vi "实时小时数据单参数上传.vi"(11 "错误输入（无错误）":errorcluster) -> (4 "数据发送起始时间":timestamp format="%<%.3X\n%Y/%m/%d>T", 15 "error out":errorcluster)   [LabVIEW 2016, in "数据传输系统.lvlib"]
uses:
  <vilib>/Utility/config.llb/Read Key (String).vi
  <vilib>/Utility/config.llb/Write Key (String).vi
  <vilib>/Utility/config.llb/NI_LVConfig.lvlib
panel:
  out "数据拆分":bool
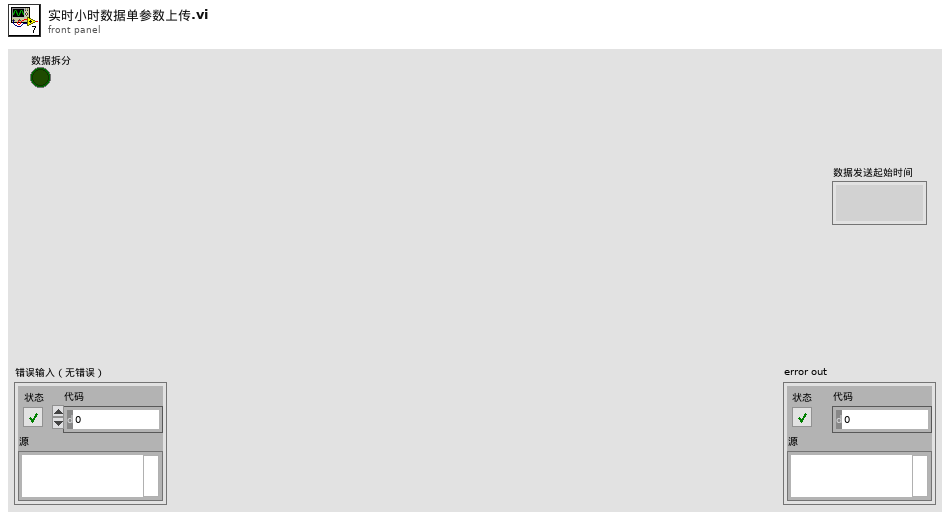
[diagram p1: front panel]
types:
  T1 = cluster{"CODMn":string, "CODCr":string, "DO":string, "铜":string, "PH":string, "氨氮":string, "比电导率":string, "水温":string, "COD":string, "浊度":string, "总氮":string, "总磷":string, "叶绿素a":string, "藻密度":string, "水位":string, "流速":string, "瞬时流量":string, "累积流量":string, "亚硝酸盐":string, "硫化物":string, "ORP":string, "铅":string, "镉":string, "锌":string, "镍":string, "锰":string, "汞":string, "气温":string, "气压":string, "风速":string, "风向":string, "盐度":string, "磷酸盐":string, "硝氮":string, "氟化物":string, "挥发酚":string, "氯化物":string, "蓝绿藻":string}
  T2 = cluster{"setini":string, "sysini":string, "hechaini":string, "actualwrite":string, "actualread":string, "datasent":string, "反控命令信息队列":string, "反控与仪器交互":string}
  T3 = typedef "NI_LVConfig.lvlib/Config Data RefNum.ctl" = refnum<k1>
  T4 = cluster{"time1":string, "time2":string, "time3":string, "time4":string, "time5":string, "time6":string, "time7":string, "time8":string, "time9":string, "time10":string, "time11":string, "time12":string, "time13":string, "time14":string, "time15":string, "time16":string, "time17":string, "time18":string, "time19":string, "time20":string, "time21":string, "time22":string, "time23":string, "time24":string, "time25":string, "time26":string, "time27":string, "time28":string, "time29":string, "time30":string, "time31":string, "time32":string, "time33":string, "time34":string, "time35":string, "time36":string, "time37":string, "time38":string}
  T5 = cluster{"水样数据索引[0]":string, "水样数据索引[1]":string, "水样数据索引[2]":string, "水样数据索引[3]":string, "水样数据索引[4]":string, "水样数据索引[5]":string, "水样数据索引[6]":string, "水样数据索引[7]":string, "水样数据索引[8]":string, "水样数据索引[9]":string, "水样数据索引[10]":string, "水样数据索引[11]":string, "水样数据索引[12]":string, "水样数据索引[13]":string, "水样数据索引[14]":string, "水样数据索引[15]":string, "水样数据索引[16]":string, "水样数据索引[17]":string, "水样数据索引[18]":string, "水样数据索引[19]":string, "水样数据索引[20]":string, "水样数据索引[21]":string, "水样数据索引[22]":string, "水样数据索引[23]":string, "水样数据索引[24]":string, "水样数据索引[25]":string, "水样数据索引[26]":string, "水样数据索引[27]":string, "水样数据索引[28]":string, "水样数据索引[29]":string, "水样数据索引[30]":string, "水样数据索引[31]":string, "水样数据索引[32]":string, "水样数据索引[33]":string, "水样数据索引[34]":string, "水样数据索引[35]":string, "水样数据索引[36]":string, "水样数据索引[37]":string}
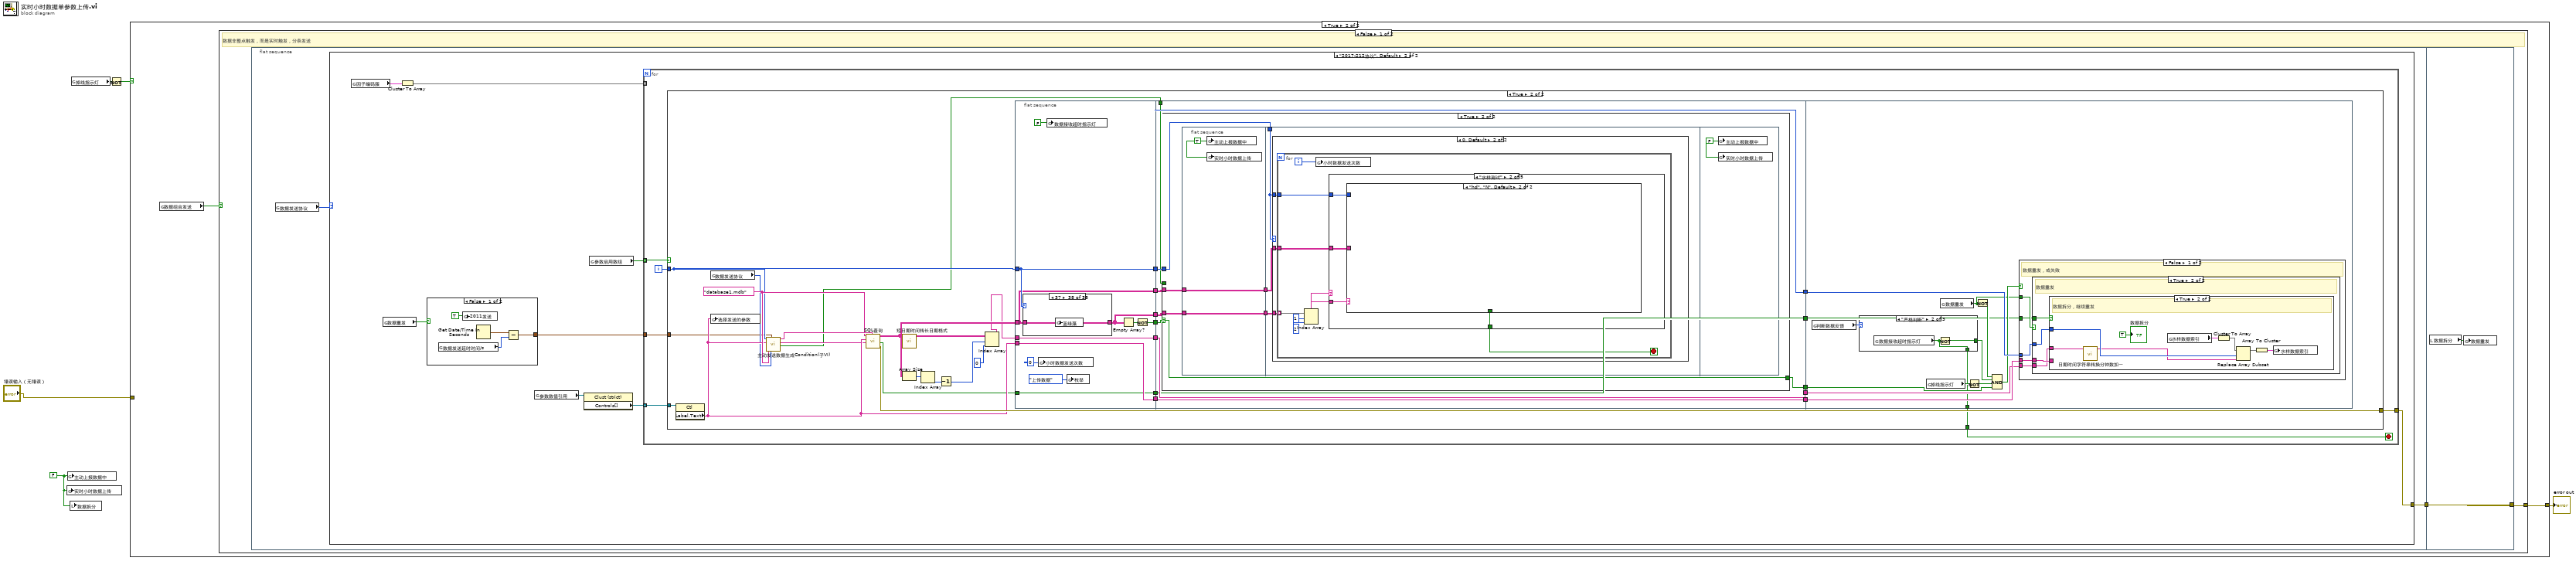
[diagram p0: block diagram]
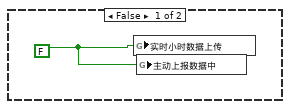
[diagram p2: hidden frame]
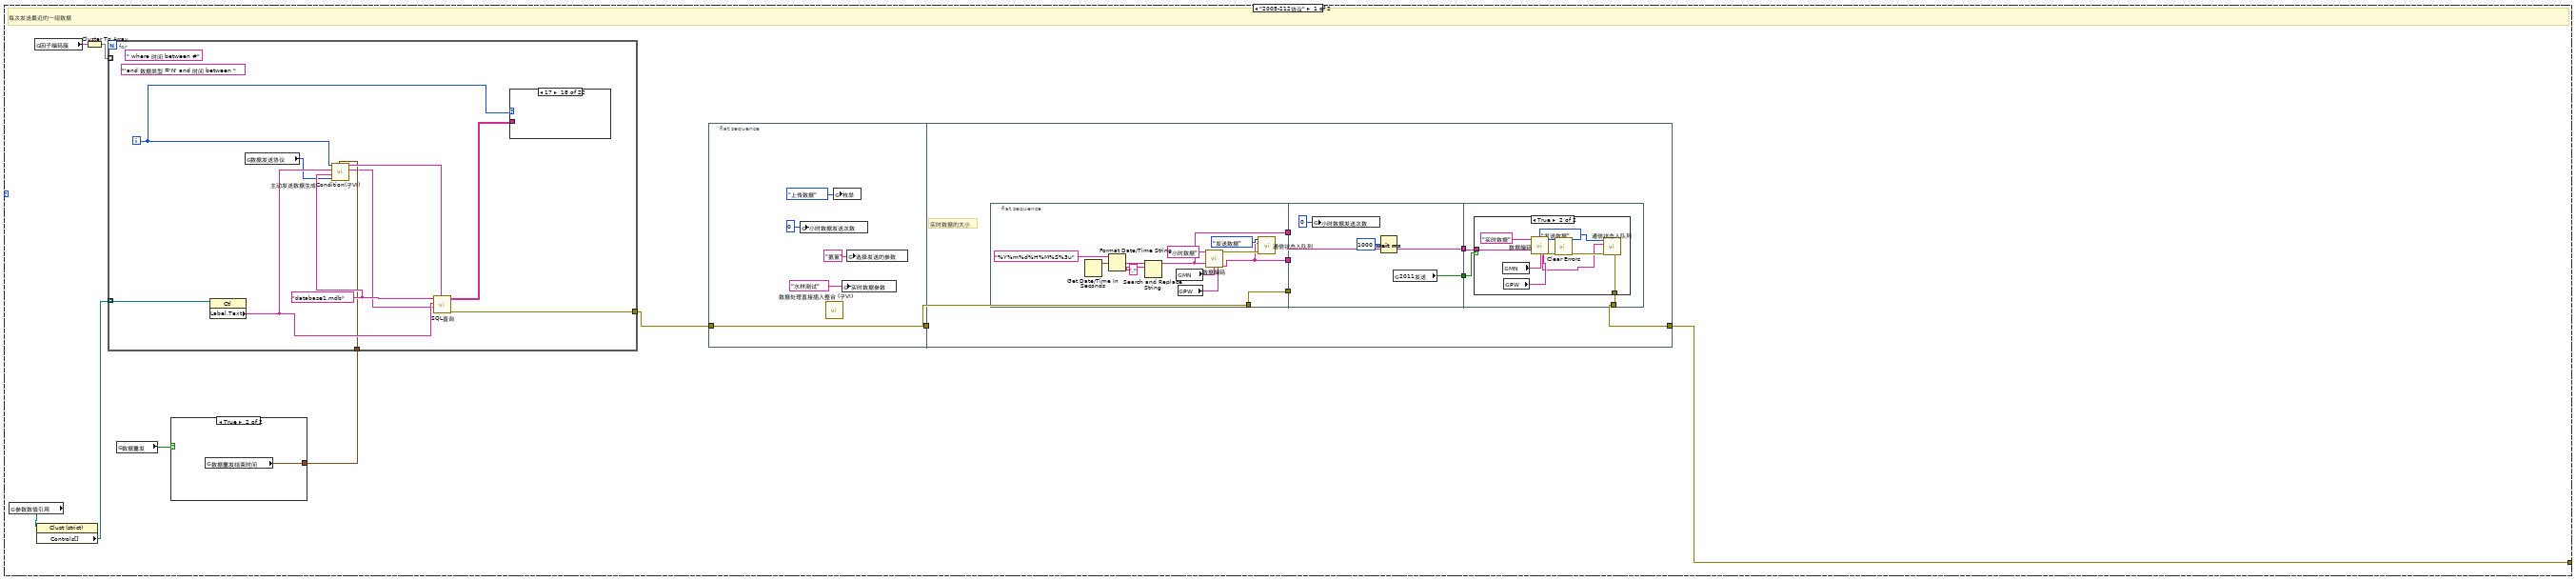
[diagram p3: hidden frame]
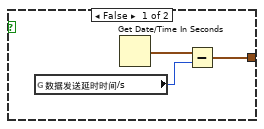
[diagram p4: hidden frame]
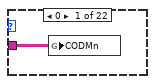
[diagram p6: hidden frame]
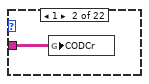
[diagram p7: hidden frame]
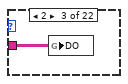
[diagram p8: hidden frame]
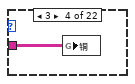
[diagram p9: hidden frame]
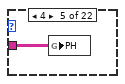
[diagram p10: hidden frame]
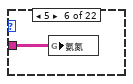
[diagram p11: hidden frame]
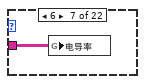
[diagram p12: hidden frame]
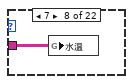
[diagram p13: hidden frame]
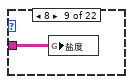
[diagram p14: hidden frame]
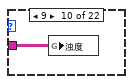
[diagram p15: hidden frame]
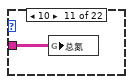
[diagram p16: hidden frame]
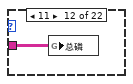
[diagram p17: hidden frame]
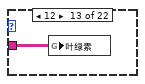
[diagram p18: hidden frame]
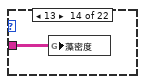
[diagram p19: hidden frame]
diagram:
  w1 = FALSE ("小时数据上传")
  n1 = global write "全局1.vi" "实时小时数据上传"(w1) -> ()
  n2 = global write "全局 数据发送重叠.vi" "主动上报数据中"(w1) -> ()
  n3 = local write "数据拆分"(w1) -> ()
  n4 = global read "全局 数据发送重叠.vi" "掉线指示灯"() -> (w5:bool)
  n5 = Not(x=w5) -> (.not. x?=w4:bool)
  n6 = case shown="True" w4 {
    tunnel: [_ w8] -> w3
    tunnel: "错误输入（无错误）" -> [_ _]
    frame False {
      w6 = FALSE ("小时数据上传")
      n7 = global write "全局1.vi" "实时小时数据上传"(w6) -> ()
      n8 = global write "全局 数据发送重叠.vi" "主动上报数据中"(w6) -> ()
    }
    frame True {
      n9 = global read "断电保存全局.vi" "数据组合发送"() -> (w7:bool)
      n10 = case shown="False" w7 {
        tunnel: [w9 _] -> w8
        frame False {
          # "数据非整点触发，而是实时触发，分条发送"
          n11 = flat-sequence {
            tunnel: [w12] -> w10
            tunnel: [w371] -> w9
            tunnel: w10 -> [w371]
            frame #0 {
              n12 = global read "断电保存全局.vi" "数据发送协议"() -> (w11:enum16{"2005-212协议", "2017-212协议"})
              n13 = case shown="\"2017-212协议\", Default" w11 {
                tunnel: [w17 w99] -> w12
                frame "2005-212协议" {
                  # "每次发送最近的一组数据"
                  n14 = global read "断电保存全局.vi" "参数数值引用"() -> (w15:refnum<vi>)
                  n15 = global read "断电保存全局.vi" "因子编码簇"() -> (w16:T1)
                  n16 = property class="Clust (strict)"(reference=w15) -> ("Controls[]"=w18:refnum<vi>[])  [unwired: 1 in, 2 out]
                  n17 = Cluster To Array(cluster=w16) -> (array=w21:string[])
                  n18 = global read "断电保存全局.vi" "数据重发"() -> (w14:bool)
                  n19 = case shown="True" w14 {
                    tunnel: [w22 w25] -> w13
                    frame False {
                      n20 = global read "断电保存全局.vi" "数据发送延时时间/s"() -> (w23:i32)
                      n21 = Get Date/Time In Seconds() -> (seconds since 1Jan1904=w24:timestamp)
                      n22 = Subtract(x=w24, y=w23) -> (x-y=w22:timestamp)
                    }
                    frame True {
                      n23 = global read "断电保存全局.vi" "数据重发结束时间"() -> (w25:timestamp)
                    }
                  }
                  n24 = for {
                    tunnel: w21 -> [_] mode=indexing
                    tunnel: [w75] -> w20
                    tunnel: w18 -> [w70] mode=indexing
                    tunnel: w13 -> [w67]
                    i -> [w68]
                    (unwired) " where 时间 between #"
                    w73 = "database1.mdb" ("database")
                    (unwired) "'and 数据类型 ='N' and 时间 between "
                    n25 = property class="Ctl"(reference=w70) -> ("Label.Text"=w74:string)  [unwired: 1 in, 2 out]
                    n26 = global read "断电保存全局.vi" "数据发送协议"() -> (w71:enum16{"2005-212协议", "2017-212协议"})
                    n27 = call "主动发送数据生成Condition(子VI).vi"("结束时间"=w67, "数据发送协议"=w71, "database"=w73, "Label.Text"=w74, "数值"=w68) -> ("columns"=w66:string[], "CONDITION"=w72:string)  [unwired: 3 in, 2 out]
                    n28 = call "SQL查询.vi"("condition"=w72, "columns"=w66, "table输入"=w74, "database"=w73) -> ("error out"=w75:errorcluster, "data"=w69:string[][])  [unwired: 4 in, 2 out]
                    n29 = case shown="17" w68 {
                      tunnel: w69 -> [w76 w77 w78 w79 w80 w81 w82 w83 w84 w85 w86 w87 w88 w89 _ _ _ _ w90 w91 w92 _]
                      frame 0 {
                        n30 = global write "全局 所有参数.vi" "CODMn"(w76) -> ()
                      }
                      frame 1 {
                        n31 = global write "全局 所有参数.vi" "CODCr"(w77) -> ()
                      }
                      frame 2 {
                        n32 = global write "全局 所有参数.vi" "DO"(w78) -> ()
                      }
                      frame 3 {
                        n33 = global write "全局 所有参数.vi" "铜"(w79) -> ()
                      }
                      frame 4 {
                        n34 = global write "全局 所有参数.vi" "PH"(w80) -> ()
                      }
                      frame 5 {
                        n35 = global write "全局 所有参数.vi" "氨氮"(w81) -> ()
                      }
                      frame 6 {
                        n36 = global write "全局 所有参数.vi" "电导率"(w82) -> ()
                      }
                      frame 7 {
                        n37 = global write "全局 所有参数.vi" "水温"(w83) -> ()
                      }
                      frame 8 {
                        n38 = global write "全局 所有参数.vi" "盐度"(w84) -> ()
                      }
                      frame 9 {
                        n39 = global write "全局 所有参数.vi" "浊度"(w85) -> ()
                      }
                      frame 10 {
                        n40 = global write "全局 所有参数.vi" "总氮"(w86) -> ()
                      }
                      frame 11 {
                        n41 = global write "全局 所有参数.vi" "总磷"(w87) -> ()
                      }
                      frame 12 {
                        n42 = global write "全局 所有参数.vi" "叶绿素"(w88) -> ()
                      }
                      frame 13 {
                        n43 = global write "全局 所有参数.vi" "藻密度"(w89) -> ()
                      }
                      frame 14 {
                      }
                      frame 15 {
                      }
                      frame 16 {
                      }
                      frame 17 {
                      }
                      frame 18 {
                        n44 = global write "全局 所有参数.vi" "亚硝酸盐"(w90) -> ()
                      }
                      frame 19 {
                        n45 = global write "全局 所有参数.vi" "硫化物"(w91) -> ()
                      }
                      frame 20 {
                        n46 = global write "全局 所有参数.vi" "ORP"(w92) -> ()
                      }
                      frame 21, Default {
                      }
                    }
                  }
                  n47 = flat-sequence {
                    tunnel: w20 -> [w26]
                    tunnel: [w26] -> w19
                    tunnel: w19 -> [w35]
                    tunnel: [w34] -> w17
                    frame #0 {
                      n48 = global write "全局 小时数据发送次数.vi" "小时数据发送次数"(0 ("小时数据发送次数")) -> ()
                      n49 = call "数据处理直接插入整合 (子VI).vi"() -> ()  [unwired: 12 in]
                      n50 = global write "全局1.vi" "枚举"(enum16{"返回请求应答", "上传数据", "返回执行结果"}."上传数据" ("枚举")) -> ()
                      n51 = global write "全局 实时数据参数.vi" "实时数据参数"("水样测试" ("实时数据参数")) -> ()
                      n52 = global write "全局 水样时间.vi" "选择发送的参数"("氨氮" ("选择发送的参数")) -> ()
                    }
                    frame #1 {
                      # "实时数据的大小"
                      n53 = flat-sequence {
                        tunnel: [w38] -> w37
                        tunnel: [w41] -> w36
                        tunnel: w35 -> [w41]
                        tunnel: [w40] -> w33
                        tunnel: w37 -> [_]
                        tunnel: w36 -> [_]
                        tunnel: w33 -> [w51]
                        tunnel: [w51] -> w32
                        tunnel: [w50] -> w31
                        tunnel: [w56] -> w34
                        tunnel: w32 -> [w55]
                        tunnel: w31 -> [w54]
                        frame #0 {
                          n54 = Get Date/Time In Seconds() -> (seconds since 1Jan1904=w47:timestamp)
                          n55 = Format Date/Time String(time format string (%c)="%Y%m%d%H%M%S%3u" ("时间格式字符串(%c)"), seconds (now)=w47) -> (date/time string=w48:string)  [unwired: 1 in]
                          n56 = Search and Replace String(input string=w48, search string="." ("搜索字符串")) -> (result string=w40:string)  [unwired: 6 in, 3 out]
                          n57 = global read "断电保存全局.vi" "MN"() -> (w44:string)
                          n58 = global read "断电保存全局.vi" "PW"() -> (w43:string)
                          n59 = call "数据编码.vi"("table输入"="小时数据" ("新元素/子数组"), "QN"=w40, "MN"=w44, "PW"=w43) -> ("错误常量"=w42:errorcluster, "通讯包字符串"=w38:string)  [unwired: 10 in]
                          n60 = call "通信状态入队列.vi"("错误输入（无错误）"=w42, "发送报文"=w38, "枚举"=enum16{"打开连接", "发送数据", "读取数据", "数据处理", "关闭连接"}."发送数据") -> ()  [unwired: 8 in, 1 out]
                        }
                        frame #1 {
                          n61 = global write "全局 小时数据发送次数.vi" "小时数据发送次数"(0 ("小时数据发送次数")) -> ()
                          n62 = Wait (ms)(milliseconds to wait=u32 1000 ("等待时间（毫秒）")) -> ()  [unwired: 1 out]
                          n63 = global read "断电保存全局.vi" "2011发送"() -> (w50:bool)
                        }
                        frame #2 {
                          n64 = case shown="True" w54 {
                            tunnel: [_ w61] -> w56
                            tunnel: w55 -> [_ w60]
                            frame False {
                            }
                            frame True {
                              n65 = global read "断电保存全局.vi" "MN"() -> (w63:string)
                              n66 = global read "断电保存全局.vi" "PW"() -> (w64:string)
                              n67 = call "数据编码.vi"("table输入"="实时数据" ("新元素/子数组"), "QN"=w60, "MN"=w63, "PW"=w64) -> ("错误常量"=w62:errorcluster, "通讯包字符串"=w57:string)  [unwired: 10 in]
                              n68 = call <vilib>:"Clear Errors.vi"("error in (no error)"=w62) -> ("error out"=w59:errorcluster)  [unwired: 5 in, 1 out]
                              n69 = call "通信状态入队列.vi"("错误输入（无错误）"=w59, "发送报文"=w57, "枚举"=enum16{"打开连接", "发送数据", "读取数据", "数据处理", "关闭连接"}."发送数据") -> ("错误输出"=w61:errorcluster)  [unwired: 8 in]
                            }
                          }
                        }
                      }
                    }
                  }
                }
                frame "2017-212协议", Default {
                  n70 = global read "断电保存全局.vi" "因子编码簇"() -> (w97:T1)
                  n71 = global read "断电保存全局.vi" "数据重发"() -> (w94:bool)
                  n72 = Cluster To Array(cluster=w97) -> (array=w100:string[])
                  n73 = case shown="False" w94 {
                    tunnel: [w102 w105] -> w93
                    frame False {
                      n74 = global read "断电保存全局.vi" "数据发送延时时间/s"() -> (w103:i32)
                      n75 = global write "断电保存全局.vi" "2011发送"(TRUE ("2011发送")) -> ()
                      n76 = Get Date/Time In Seconds() -> (seconds since 1Jan1904=w104:timestamp)
                      n77 = Subtract(x=w104, y=w103) -> (x-y=w102:timestamp)
                    }
                    frame True {
                      n78 = global read "断电保存全局.vi" "数据重发结束时间"() -> (w105:timestamp)
                    }
                  }
                  n79 = global read "断电保存全局.vi" "参数数值引用"() -> (w96:refnum<vi>)
                  n80 = property class="Clust (strict)"(reference=w96) -> ("Controls[]"=w98:refnum<vi>[])  [unwired: 1 in, 2 out]
                  n81 = global read "断电保存全局.vi" "参数启用数组"() -> (w95:bool[])
                  n82 = for {
                    tunnel: w100 -> [_] mode=indexing
                    tunnel: [w111] -> w99
                    tunnel: w98 -> [w109] mode=indexing
                    tunnel: w95 -> [w108] mode=indexing
                    tunnel: w93 -> [w107]
                    i -> [w110]
                    stop <- w106 stop-if-true
                    n83 = case shown="True" w108 {
                      tunnel: [_ w132] -> w111
                      tunnel: w110 -> [_ w123]
                      tunnel: w109 -> [_ w122]
                      tunnel: w107 -> [_ w119]
                      tunnel: [_ w117] -> w106
                      frame False {
                      }
                      frame True {
                        w131 = "database1.mdb" ("database")
                        n84 = property class="Ctl"(reference=w122) -> ("Label.Text"=w130:string)  [unwired: 1 in, 2 out]
                        n85 = global read "断电保存全局.vi" "数据发送协议"() -> (w129:enum16{"2005-212协议", "2017-212协议"})
                        n86 = global write "全局 水样时间.vi" "选择发送的参数"(w130) -> ()
                        n87 = call "主动发送数据生成Condition(子VI).vi"("结束时间"=w119, "数据发送协议"=w129, "database"=w131, "Label.Text"=w130, "数值"=w123) -> ("database溢出"=w112:bool, "columns"=w121:string[], "CONDITION"=w134:string)  [unwired: 3 in, 1 out]
                        n88 = call "SQL查询.vi"("condition"=w134, "columns"=w121, "table输入"=w130, "database"=w131) -> ("error out"=w132:errorcluster, "拆分数据"=w115:bool, "data"=w126:string[][])  [unwired: 4 in, 1 out]
                        n89 = call "短日期时间转长日期格式.vi"("data"=w126) -> ("输出数组"=w133:string[][])  [unwired: 10 in]
                        n90 = Array Size(array=w126) -> (size(s)=w128:i32[])
                        n91 = Index Array(array=w128) -> (element=w127:i32)  [unwired: 1 in]
                        n92 = Decrement(x=w127) -> (x-1=w125:i32)
                        n93 = Index Array(array=w133, index (row)=w125, index (col)=0 ("禁用的索引 (列)")) -> (element=w113:string)
                        n94 = flat-sequence {
                          tunnel: [w146] -> w142
                          tunnel: [w145] -> w141
                          tunnel: w126 -> [w144]
                          tunnel: w123 -> [w149]
                          tunnel: w130 -> [w151]
                          tunnel: [w151] -> w140
                          tunnel: w113 -> [w150]
                          tunnel: [w150] -> w139
                          tunnel: [w149] -> w138
                          tunnel: [w144] -> w118
                          tunnel: [w143] -> w116
                          tunnel: w115 -> [w143]
                          tunnel: w142 -> [w196]
                          tunnel: w141 -> [w200]
                          tunnel: [w199] -> w137
                          tunnel: w140 -> [w199]
                          tunnel: [w198] -> w136
                          tunnel: w139 -> [w198]
                          tunnel: [w197] -> w135
                          tunnel: w138 -> [w197]
                          tunnel: [w193] -> w120
                          tunnel: w118 -> [w195]
                          tunnel: w116 -> [w194]
                          tunnel: [w194] -> w114
                          tunnel: w112 -> [w192]
                          tunnel: w137 -> [w311]
                          tunnel: w136 -> [w310]
                          tunnel: w135 -> [w309]
                          tunnel: w120 -> [w308]
                          tunnel: [w300] -> w117
                          tunnel: w114 -> [w299]
                          frame #0 {
                            n95 = case shown="37" w149 {
                              tunnel: w144 -> [w154 w155 w156 w157 w158 w159 w160 w161 w162 w163 w164 w165 w166 w167 _ _ _ _ w172 w173 w174 w175 w176 w177 w178 w179 w180 _ _ _ _ w185 w186 w187 w188 w189 w190 w191]
                              tunnel: [w154 w155 w156 w157 w158 w159 w160 w161 w162 w163 w164 w165 w166 w167 w168 w169 w170 w171 w172 w173 w174 w175 w176 w177 w178 w179 w180 w181 w182 w183 w184 w185 w186 w187 w188 w189 w190 w191] -> w145
                              frame 0, Default {
                                n96 = global write "全局 所有参数.vi" "CODMn"(w154) -> ()
                              }
                              frame 1 {
                                n97 = global write "全局 所有参数.vi" "CODCr"(w155) -> ()
                              }
                              frame 2 {
                                n98 = global write "全局 所有参数.vi" "DO"(w156) -> ()
                              }
                              frame 3 {
                                n99 = global write "全局 所有参数.vi" "铜"(w157) -> ()
                              }
                              frame 4 {
                                n100 = global write "全局 所有参数.vi" "PH"(w158) -> ()
                              }
                              frame 5 {
                                n101 = global write "全局 所有参数.vi" "氨氮"(w159) -> ()
                              }
                              frame 6 {
                                n102 = global write "全局 所有参数.vi" "电导率"(w160) -> ()
                              }
                              frame 7 {
                                n103 = global write "全局 所有参数.vi" "水温"(w161) -> ()
                              }
                              frame 8 {
                                n104 = global write "全局 所有参数.vi" "盐度"(w162) -> ()
                              }
                              frame 9 {
                                n105 = global write "全局 所有参数.vi" "浊度"(w163) -> ()
                              }
                              frame 10 {
                                n106 = global write "全局 所有参数.vi" "总氮"(w164) -> ()
                              }
                              frame 11 {
                                n107 = global write "全局 所有参数.vi" "总磷"(w165) -> ()
                              }
                              frame 12 {
                                n108 = global write "全局 所有参数.vi" "叶绿素"(w166) -> ()
                              }
                              frame 13 {
                                n109 = global write "全局 所有参数.vi" "藻密度"(w167) -> ()
                              }
                              frame 14 {
                                n110 = global read "全局 所有参数.vi" "水位"() -> (w168:string[][])
                              }
                              frame 15 {
                                n111 = global read "全局 所有参数.vi" "流速"() -> (w169:string[][])
                              }
                              frame 16 {
                                n112 = global read "全局 所有参数.vi" "瞬时流量"() -> (w170:string[][])
                              }
                              frame 17 {
                                n113 = global read "全局 所有参数.vi" "累积流量"() -> (w171:string[][])
                              }
                              frame 18 {
                                n114 = global write "全局 所有参数.vi" "亚硝酸盐"(w172) -> ()
                              }
                              frame 19 {
                                n115 = global write "全局 所有参数.vi" "硫化物"(w173) -> ()
                              }
                              frame 20 {
                                n116 = global write "全局 所有参数.vi" "ORP"(w174) -> ()
                              }
                              frame 21 {
                                n117 = global write "全局 所有参数.vi" "铅"(w175) -> ()
                              }
                              frame 22 {
                                n118 = global write "全局 所有参数.vi" "镉"(w176) -> ()
                              }
                              frame 23 {
                                n119 = global write "全局 所有参数.vi" "锌"(w177) -> ()
                              }
                              frame 24 {
                                n120 = global write "全局 所有参数.vi" "镍"(w178) -> ()
                              }
                              frame 25 {
                                n121 = global write "全局 所有参数.vi" "锰"(w179) -> ()
                              }
                              frame 26 {
                                n122 = global write "全局 所有参数.vi" "汞"(w180) -> ()
                              }
                              frame 27 {
                                n123 = global read "全局 所有参数.vi" "气温"() -> (w181:string[][])
                              }
                              frame 28 {
                                n124 = global read "全局 所有参数.vi" "气压"() -> (w182:string[][])
                              }
                              frame 29 {
                                n125 = global read "全局 所有参数.vi" "风速"() -> (w183:string[][])
                              }
                              frame 30 {
                                n126 = global read "全局 所有参数.vi" "风向"() -> (w184:string[][])
                              }
                              frame 31 {
                                n127 = global write "全局 所有参数.vi" "盐度 2"(w185) -> ()
                              }
                              frame 32 {
                                n128 = global write "全局 所有参数.vi" "磷酸盐"(w186) -> ()
                              }
                              frame 33 {
                                n129 = global write "全局 所有参数.vi" "硝氮"(w187) -> ()
                              }
                              frame 34 {
                                n130 = global write "全局 所有参数.vi" "氟化物"(w188) -> ()
                              }
                              frame 35 {
                                n131 = global write "全局 所有参数.vi" "挥发酚"(w189) -> ()
                              }
                              frame 36 {
                                n132 = global write "全局 所有参数.vi" "氯化物"(w190) -> ()
                              }
                              frame 37 {
                                n133 = global write "全局 所有参数.vi" "蓝绿藻"(w191) -> ()
                              }
                            }
                            n134 = global write "全局 小时数据发送次数.vi" "小时数据发送次数"(0 ("小时数据发送次数")) -> ()
                            n135 = global write "全局 数据发送重叠.vi" "数据接收超时指示灯"(FALSE ("数据接收超时指示灯")) -> ()
                            n136 = global write "全局1.vi" "枚举"(enum16{"返回请求应答", "上传数据", "返回执行结果"}."上传数据" ("枚举")) -> ()
                            n137 = Empty Array?(array=w145) -> (empty?=w147:bool)
                            n138 = Not(x=w147) -> (.not. x?=w146:bool)
                          }
                          frame #1 {
                            n139 = case shown="True" w196 {
                              selector: w196 -> [_ w202]
                              tunnel: w200 -> [_ w207]
                              tunnel: w197 -> [_ w206]
                              tunnel: w195 -> [_ w204]
                              tunnel: [w201 w202] -> w193
                              tunnel: w192 -> [w201 _]
                              frame False {
                              }
                              frame True {
                                n140 = flat-sequence {
                                tunnel: w207 -> [w210]
                                tunnel: [w210] -> w205
                                tunnel: w204 -> [w208]
                                tunnel: [w208] -> w203
                                tunnel: w206 -> [w212]
                                tunnel: w205 -> [w213]
                                tunnel: w203 -> [w211]
                                frame #0 {
                                w209 = TRUE ("小时数据上传")
                                n141 = global write "全局 数据发送重叠.vi" "主动上报数据中"(w209) -> ()
                                n142 = global write "全局1.vi" "实时小时数据上传"(w209) -> ()
                                }
                                frame #1 {
                                n143 = case shown="0, Default" w212 {
                                selector: w212 -> [w214 _]
                                tunnel: w212 -> [_ w245]
                                tunnel: w213 -> [w217 w244]
                                tunnel: w211 -> [w216 w243]
                                frame 14..17, 27..30 {
                                n144 = for {
                                tunnel: [w241] -> w218
                                tunnel: w214 -> [w240]
                                tunnel: w217 -> [_] mode=indexing
                                i -> [w242]
                                stop <- w239 stop-if-true
                                n145 = call "小时数据发送 (子VI).vi"("数值"=w240) -> ("error out"=w241:errorcluster, "超时退出"=w239:bool)  [unwired: 9 in]
                                n146 = global write "全局 小时数据发送次数.vi" "小时数据发送次数"(w242) -> ()
                                }
                                n147 = global read "断电保存全局.vi" "2011发送"() -> (w215:bool)
                                n148 = case shown="True" w215 {
                                tunnel: w218 -> [_ w223]
                                tunnel: w214 -> [_ w222]
                                tunnel: w216 -> [_ w221]
                                tunnel: w214 -> [_ w219]
                                frame False {
                                }
                                frame True {
                                n149 = flat-sequence {
                                tunnel: w223 -> [w227]
                                tunnel: [w227] -> w224
                                tunnel: w222 -> [w226]
                                tunnel: w221 -> [w225]
                                tunnel: [w225] -> w220
                                frame #0 {
                                n150 = case shown="30" w226 {
                                tunnel: w225 -> [_ w228 w229 w230 w231 w232 w233 w234 w235]
                                frame 0, Default {
                                }
                                frame 14 {
                                n151 = global write "全局 所有参数.vi" "水位"(w228) -> ()
                                }
                                frame 15 {
                                n152 = global write "全局 所有参数.vi" "流速"(w229) -> ()
                                }
                                frame 16 {
                                n153 = global write "全局 所有参数.vi" "瞬时流量"(w230) -> ()
                                }
                                frame 17 {
                                n154 = global write "全局 所有参数.vi" "累积流量"(w231) -> ()
                                }
                                frame 27 {
                                n155 = global write "全局 所有参数.vi" "气温"(w232) -> ()
                                }
                                frame 28 {
                                n156 = global write "全局 所有参数.vi" "气压"(w233) -> ()
                                }
                                frame 29 {
                                n157 = global write "全局 所有参数.vi" "风速"(w234) -> ()
                                }
                                frame 30 {
                                n158 = global write "全局 所有参数.vi" "风向"(w235) -> ()
                                }
                                }
                                }
                                }
                                n159 = for {
                                tunnel: w224 -> [_]
                                tunnel: w220 -> [_] mode=indexing
                                tunnel: w219 -> [w237]
                                i -> [w238]
                                stop <- w236 stop-if-true
                                n160 = global write "全局 小时数据发送次数.vi" "小时数据发送次数"(w238) -> ()
                                n161 = call "实时数据发送 (子VI).vi"("数值"=w237) -> ("超时退出"=w236:bool)  [unwired: 10 in]
                                }
                                }
                                }
                                }
                                frame 0, Default {
                                n162 = for {
                                tunnel: w245 -> [w248]
                                tunnel: w244 -> [w254] mode=indexing
                                tunnel: w243 -> [w250]
                                i -> [w249]
                                stop <- w246 stop-if-true
                                n163 = Index Array(array=w254, index #1=1 ("索引"), index #2=2 ("索引")) -> (element #1=w247:string, element #2=w251:string)
                                n164 = global write "全局 小时数据发送次数.vi" "小时数据发送次数"(w249) -> ()
                                n165 = case shown="\"水样测试\"" w247 {
                                tunnel: w248 -> [_ w258 _ _ _]
                                tunnel: w251 -> [_ w257 w290 w293 w296]
                                tunnel: w250 -> [_ w256 _ _ _]
                                tunnel: [_ w255 w289 w292 w295] -> w246
                                frame "假", Default {
                                }
                                frame "水样测试" {
                                n166 = case shown="\"hd\", \"N\", Default" w257 {
                                tunnel: w258 -> [w262 w283]
                                tunnel: w256 -> [w261 w282]
                                tunnel: [w259 w280] -> w255
                                frame "M" {
                                n167 = global read "断电保存全局.vi" "2011发送"() -> (w260:bool)
                                n168 = case shown="True" w260 {
                                tunnel: w262 -> [_ w265]
                                tunnel: w261 -> [_ w264]
                                tunnel: [_ w263] -> w259
                                frame False {
                                }
                                frame True {
                                n169 = flat-sequence {
                                tunnel: w265 -> [w267]
                                tunnel: w264 -> [w268]
                                tunnel: [w267] -> w266
                                tunnel: w266 -> [w278]
                                tunnel: [w277] -> w263
                                frame #0 {
                                n170 = case shown="14" w267 {
                                tunnel: w268 -> [_ w269 w270 w271 w272 w273 w274 w275 w276]
                                frame 0, Default {
                                }
                                frame 14 {
                                n171 = global write "全局 所有参数.vi" "水位"(w269) -> ()
                                }
                                frame 15 {
                                n172 = global write "全局 所有参数.vi" "流速"(w270) -> ()
                                }
                                frame 16 {
                                n173 = global write "全局 所有参数.vi" "瞬时流量"(w271) -> ()
                                }
                                frame 17 {
                                n174 = global write "全局 所有参数.vi" "累积流量"(w272) -> ()
                                }
                                frame 27 {
                                n175 = global write "全局 所有参数.vi" "气温"(w273) -> ()
                                }
                                frame 28 {
                                n176 = global write "全局 所有参数.vi" "气压"(w274) -> ()
                                }
                                frame 29 {
                                n177 = global write "全局 所有参数.vi" "风速"(w275) -> ()
                                }
                                frame 30 {
                                n178 = global write "全局 所有参数.vi" "风向"(w276) -> ()
                                }
                                }
                                }
                                frame #1 {
                                n179 = call "实时数据发送 (子VI).vi"("数值"=w278) -> ("超时退出"=w277:bool)  [unwired: 10 in]
                                }
                                }
                                }
                                }
                                }
                                frame "hd", "N", Default {
                                n180 = call "小时数据发送 (子VI).vi"("数值"=w283) -> ("error out"=w281:errorcluster, "超时退出"=w279:bool)  [unwired: 9 in]
                                n181 = global read "断电保存全局.vi" "2011发送"() -> (w284:bool)
                                n182 = case shown="True" w284 {
                                tunnel: w283 -> [_ w288]
                                tunnel: w282 -> [_ _]
                                tunnel: w281 -> [_ _]
                                tunnel: [_ w285] -> w280
                                tunnel: w279 -> [_ w287]
                                frame False {
                                }
                                frame True {
                                n183 = call "实时数据发送 (子VI).vi"("数值"=w288) -> ("超时退出"=w286:bool)  [unwired: 10 in]
                                n184 = Or(x=w287, y=w286) -> (x .or. y?=w285:bool)
                                }
                                }
                                }
                                }
                                }
                                frame "空白测试", "零点核查" {
                                n185 = case shown="\"N\", Default" w290 {
                                tunnel: [_ w291] -> w289
                                frame "M" {
                                }
                                frame "N", Default {
                                n186 = call "零点核查数据发送 (子VI).vi"() -> ("超时退出"=w291:bool)  [unwired: 11 in]
                                }
                                }
                                }
                                frame "跨度核查" {
                                n187 = case shown="\"N\", Default" w293 {
                                tunnel: [_ w294] -> w292
                                frame "M" {
                                }
                                frame "N", Default {
                                n188 = call "跨度核查数据发送 (子VI).vi"() -> ("超时退出"=w294:bool)  [unwired: 11 in]
                                }
                                }
                                }
                                frame "标样核查" {
                                n189 = case shown="\"N\", Default" w296 {
                                tunnel: [_ w297] -> w295
                                frame "M" {
                                }
                                frame "N", Default {
                                n190 = call "标样核查数据发送(子VI).vi"() -> ("超时退出"=w297:bool)  [unwired: 11 in]
                                }
                                }
                                }
                                }
                                }
                                }
                                }
                                }
                                frame #2 {
                                w298 = FALSE ("小时数据上传")
                                n191 = global write "全局 数据发送重叠.vi" "主动上报数据中"(w298) -> ()
                                n192 = global write "全局1.vi" "实时小时数据上传"(w298) -> ()
                                }
                                }
                              }
                            }
                          }
                          frame #2 {
                            n193 = global read "断电保存全局.vi" "判断数据反馈"() -> (w305:enum16{"非严格判断", "严格判断", "不判断"})
                            n194 = case shown="\"严格判断\"" w305 {
                              tunnel: [TRUE w315 TRUE] -> w304
                              tunnel: [FALSE ("数据接收超时指示灯") w314 FALSE ("数据接收超时指示灯")] -> w300
                              frame "非严格判断", Default {
                              }
                              frame "严格判断" {
                                n195 = global read "全局 数据发送重叠.vi" "数据接收超时指示灯"() -> (w314:bool)
                                n196 = Not(x=w314) -> (.not. x?=w315:bool)
                              }
                              frame "不判断" {
                              }
                            }
                            n197 = global read "全局 数据发送重叠.vi" "掉线指示灯"() -> (w307:bool)
                            n198 = global read "断电保存全局.vi" "数据重发"() -> (w301:bool)
                            n199 = Not(x=w307) -> (.not. x?=w306:bool)
                            n200 = Not(x=w301) -> (.not. x?=w302:bool)
                            n201 = Compound Arithmetic op=AND ("复合运算")(w302, w304, w306, w308) -> (w303:bool)
                            n202 = case shown="False" w303 {
                              tunnel: w310 -> [w318 w361]
                              tunnel: w309 -> [w320 w355]
                              tunnel: w311 -> [w322 w362]
                              tunnel: w301 -> [w321 _]
                              tunnel: w299 -> [w319 _]
                              frame False {
                                # "数据重发，或失败"
                                n203 = case shown="True" w321 {
                                tunnel: w322 -> [_ w326]
                                tunnel: w320 -> [_ w325]
                                tunnel: w319 -> [_ w324]
                                tunnel: w318 -> [_ w323]
                                frame False {
                                # "数据发送失败"
                                }
                                frame True {
                                # "数据重发"
                                n204 = case shown="True" w324 {
                                tunnel: w326 -> [w330 _]
                                tunnel: w325 -> [w328 w344]
                                tunnel: w323 -> [_ w345]
                                frame False {
                                # "重发完成恢复本地数据时间"
                                n205 = global read "全局1.vi" "配置文件队列名"() -> (w327:T2)
                                n206 = Unbundle By Name(w327) -> ("setini"=w337:string)
                                n207 = call <vilib>:"Application Directory.vi"() -> ("Application Directory"=w331:path)
                                n208 = Build Path(base path=w331, name or relative path=w337) -> (appended path=w332:path)
                                n209 = call <vilib>:"Open Config Data.vi"("configuration file path"=w332) -> ("error out"=w338:errorcluster, "refnum"=w333:T3)  [unwired: 8 in, 1 out]
                                n210 = global read "全局 水样时间.vi" "水样数据索引"() -> (w339:T4)
                                n211 = call-poly <vilib>:"Read Key.vi"("section"="线程一数据搜索起始时间", "error in (no error)"=w338, "key"=w330, "refnum"=w333) -> ("error out"=w336:errorcluster, "value"=w329:string, "refnum out"=w335:T3)  [unwired: 4 in, 1 out]
                                n212 = Cluster To Array(cluster=w339) -> (array=w340:string[])
                                n213 = call <vilib>:"Close Config Data.vi"("error in (no error)"=w336, "refnum"=w335) -> ()  [unwired: 8 in, 2 out]
                                n214 = Replace Array Subset(array=w340, new element=w329, index=w328) -> (w341:string[])
                                n215 = Array To Cluster(array=w341) -> (cluster=w342:T5)
                                n216 = global write "全局 水样时间.vi" "水样数据索引"(w342) -> ()
                                }
                                frame True {
                                # "数据拆分，继续重发"
                                n217 = call "日期时间字符串转换分钟数加一.vi"("data[0]"=w345) -> ("日期/时间字符串"=w343:string)  [unwired: 10 in]
                                n218 = global read "全局 水样时间.vi" "水样数据索引"() -> (w346:T4)
                                n219 = Cluster To Array(cluster=w346) -> (array=w347:string[])
                                n220 = Replace Array Subset(array=w347, new element=w343, index=w344) -> (w348:string[])
                                n221 = Array To Cluster(array=w348) -> (cluster=w349:T5)
                                n222 = global write "全局 水样时间.vi" "水样数据索引"(w349) -> ()
                                "数据拆分" <- TRUE
                                }
                                }
                                }
                                }
                              }
                              frame True {
                                # "保存本地"
                                n223 = global read "全局1.vi" "配置文件队列名"() -> (w351:T2)
                                n224 = call "日期时间字符串转换分钟数加一.vi"("枚举"=enum16{"分钟数加一", "秒数加一", "小时数加一"}."秒数加一", "data[0]"=w361) -> ("日期/时间字符串"=w354:string)  [unwired: 9 in]
                                n225 = Unbundle By Name(w351) -> ("setini"=w352:string)
                                n226 = global read "全局 水样时间.vi" "水样数据索引"() -> (w356:T4)
                                n227 = call <vilib>:"Application Directory.vi"() -> ("Application Directory"=w363:path)
                                n228 = Build Path(base path=w363, name or relative path=w352) -> (appended path=w364:path)
                                n229 = Cluster To Array(cluster=w356) -> (array=w357:string[])
                                n230 = call <vilib>:"Open Config Data.vi"("configuration file path"=w364) -> ("error out"=w366:errorcluster, "refnum"=w365:T3)  [unwired: 8 in, 1 out]
                                n231 = call "时间日期字符串至时间标识转换.vi"("时间日期字符串"=w354) -> ("时间标识"=→"数据发送起始时间":timestamp)  [unwired: 10 in]
                                n232 = call-poly <vilib>:"Write Key.vi"("section"="线程一数据搜索起始时间", "error in (no error)"=w366, "value"=w354, "key"=w362, "refnum"=w365) -> ("error out"=w368:errorcluster, "refnum out"=w367:T3)  [unwired: 4 in, 1 out]
                                n233 = Replace Array Subset(array=w357, new element=w354, index=w355) -> (w358:string[])
                                n234 = Array To Cluster(array=w358) -> (cluster=w359:T5)
                                n235 = call <vilib>:"Close Config Data.vi"("error in (no error)"=w368, "refnum"=w367) -> ()  [unwired: 8 in, 2 out]
                                n236 = global write "全局 水样时间.vi" "水样数据索引"(w359) -> ()
                              }
                            }
                          }
                        }
                      }
                    }
                  }
                }
              }
            }
            frame #1 {
              n237 = local read "数据拆分"() -> (w370:bool)
              n238 = global write "断电保存全局.vi" "数据重发"(w370) -> ()
            }
          }
        }
        frame True {
          # "数据整点触发，整条发送"
          n239 = flat-sequence {
            frame #0 {
              n240 = global read "断电保存全局.vi" "数据发送通道"() -> (w372:enum16{"TCP", "VISA"})
              n241 = global read "断电保存全局.vi" "MN"() -> (w374:string)
              n242 = global read "断电保存全局.vi" "PW"() -> (w373:string)
              n243 = call "数据全参数一起发送整点触发.vi"("数据发送通道"=w372, "PW"=w373, "MN"=w374) -> ()  [unwired: 8 in]
            }
            frame #1 {
              w375 = FALSE ("主动上报数据中")
              n244 = global write "全局 数据发送重叠.vi" "主动上报数据中"(w375) -> ()
              n245 = global write "全局1.vi" "实时小时数据上传"(w375) -> ()
            }
          }
        }
      }
    }
  }
  "error out" <- w3
